vi "Write Dispatcher Error.vi"(8 "error in (no error)":errorcluster, 9 "timeout in ms (0)":i32 format="%d ms", 10 "error":errorcluster, 11 "Dispatcher Interface in":refnum<class "Dispatcher Interface.lvclass">) -> (0 "error out":errorcluster, 3 "Dispatcher Interface out":refnum<class "Dispatcher Interface.lvclass">)   [LabVIEW 2021, in "DSF Core.lvlib" / "Dispatcher Interface.lvclass"]
uses:
  Dispatcher Interface.lvclass
  C:/dev/git/custom-devices/niveristand-data-sharing-framework-custom-device/Source/Core/Classes/Interface/Interface.lvclass
  Interface.lvclass/Interface.ctl
  Write RT FIFO.vi
  Error Timeout.vi
  Interface.lvclass
  C:/dev/git/custom-devices/niveristand-data-sharing-framework-custom-device/Source/Core/Classes/Interface/Dispatcher/Dispatcher Interface.lvclass
  DSF Core.lvlib
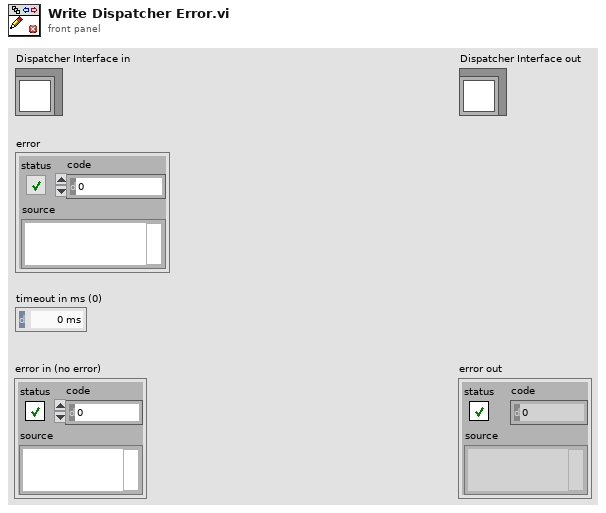
[diagram p1: front panel]
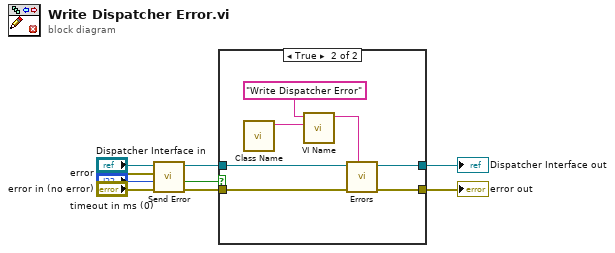
[diagram p0: block diagram]
diagram:
  n1 = call "Send Error.vi"("error in (no error)"="error in (no error)", "timeout in ms (0)"="timeout in ms (0)", "error"="error", "Interface in"="Dispatcher Interface in") -> ("error out"=w4:errorcluster, "timed out?"=w3:bool, "Interface out"=w5:refnum<class "Dispatcher Interface.lvclass">)  [unwired: 4 in, 1 out]
  n2 = case shown="True" w3 {
    tunnel: w4 -> [w10 w17]
    tunnel: w5 -> [w11 w18]
    tunnel: [w11 w16] -> w2
    tunnel: [w10 w15] -> w1
    frame False {
    }
    frame True {
      n3 = call "Class Name.vi"() -> ("class name"=w14:string)  [unwired: 11 in]
      n4 = call "VI Name.vi"("class name (\"\")"=w14, "vi name"="Write Dispatcher Error" ("error source vi name")) -> ("full VI name"=w12:string)  [unwired: 9 in]
      n5 = call-poly "Errors.vi"("error source vi name"=w12, "error in (no error)"=w17, "Interface in"=w18) -> ("error out"=w15:errorcluster, "Interface out"=w16:refnum<class "Dispatcher Interface.lvclass">)  [unwired: 7 in]
    }
  }
  "error out" <- w1
  "Dispatcher Interface out" <- w2
